vi "ErrorMessage.vi"(0 "VisaCluster":T1, 5 "Message In":string, 11 "error in (no error)":errorcluster) -> (4 "VisaCluster":T1, 6 "Message Out":string, 15 "error out":errorcluster)   [LabVIEW 2014, in "FH 55.lvlib"]
doc: "Dieses VI überprüft die Antwort aus dem Gaussmeter. Ist die Antwort leer oder enthält sie das Wort ERROR wird ein Fehler zurückgegeben.\n\nKeine Antwort: -30000\nERROR:\n parameter: -3999\n command: -4999\n sonstiger: -50000\n\n\n\nThis VI checks the answer from the gaussmeter. If the answer is empty or contains the word ERROR, an error is returned\n\nNo reply -30 000\nERROR:\n Parameters: -3999\n command: -4999\n other: -50 000"
uses:
  FH 55.lvlib
  TypeDef/VisaCluster.ctl
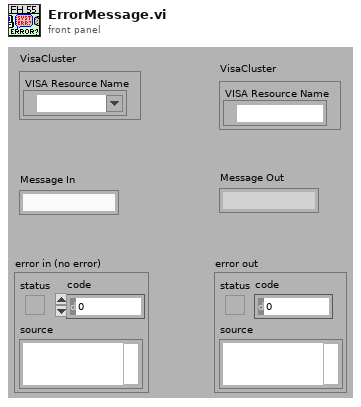
[diagram p1: front panel]
types:
  T1 = typedef "FH 55.lvlib/VisaCluster.ctl" = cluster{"VISA Resource Name":refnum<visa-resource-name>}
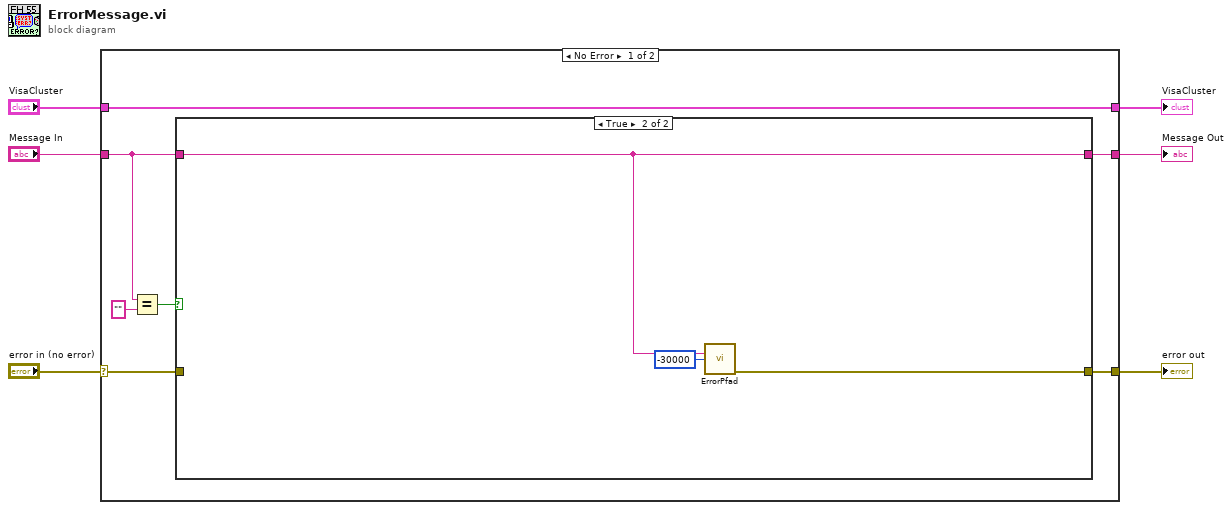
[diagram p0: block diagram]
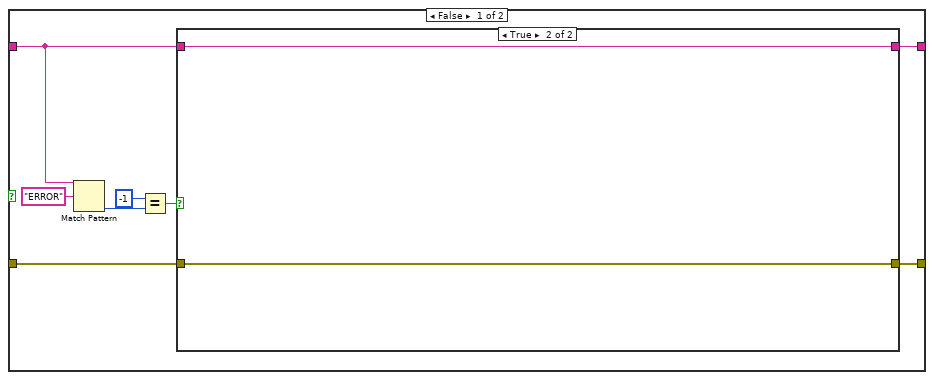
[diagram p2: hidden frame]
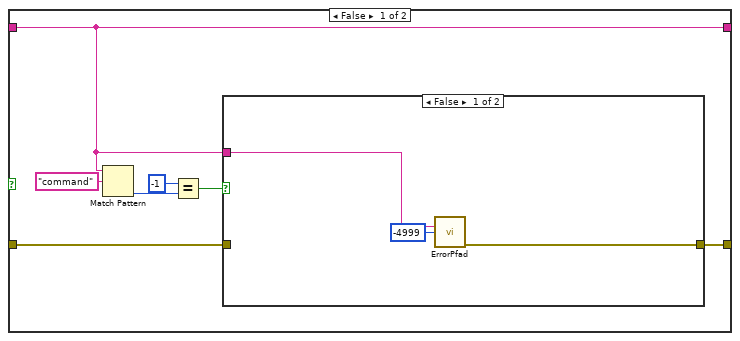
[diagram p3: hidden frame]
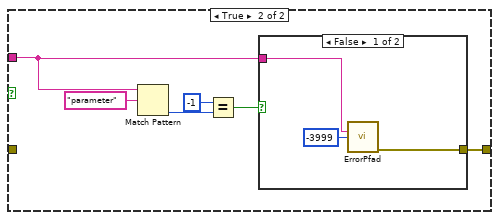
[diagram p4: hidden frame]
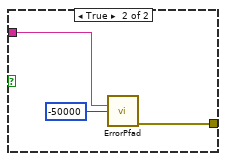
[diagram p5: hidden frame]
diagram:
  n1 = case shown="No Error" "error in (no error)" {
    selector: "error in (no error)" -> [w11 w49]
    tunnel: [w10 w49] -> w5
    tunnel: [w12 w51] -> w3
    tunnel: "VisaCluster" -> [w12 w51]
    tunnel: "Message In" -> [w9 w50]
    tunnel: [w13 w50] -> w1
    frame No Error {
      n2 = Equal?(x=w9, y="") -> (x = y?=w7:bool)
      n3 = case shown="True" w7 {
        tunnel: [w17 w48] -> w13
        tunnel: w11 -> [w16 _]
        tunnel: [w15 w47] -> w10
        tunnel: w9 -> [w14 w48]
        frame False {
          n4 = Match Pattern(string=w14, regular expression="ERROR") -> (offset past match=w20:i32)  [unwired: 1 in, 3 out]
          n5 = Equal?(x=-1, y=w20) -> (x = y?=w18:bool)
          n6 = case shown="True" w18 {
            tunnel: [w23 w44] -> w17
            tunnel: w16 -> [w22 w45]
            tunnel: [w28 w45] -> w15
            tunnel: w14 -> [w23 w44]
            frame False {
              n7 = Match Pattern(string=w23, regular expression="command") -> (offset past match=w26:i32)  [unwired: 1 in, 3 out]
              n8 = Equal?(x=-1, y=w26) -> (x = y?=w24:bool)
              n9 = case shown="False" w24 {
                tunnel: [w29 w32] -> w28
                tunnel: w23 -> [w31 w33]
                tunnel: w22 -> [_ _]
                frame False {
                  n10 = call "ErrorPfad.vi"("Message In"=w31, "Numeric"=-4999 ("code")) -> ("error out"=w29:errorcluster)  [unwired: 12 in, 1 out]
                }
                frame True {
                  n11 = Match Pattern(string=w33, regular expression="parameter") -> (offset past match=w36:i32)  [unwired: 1 in, 3 out]
                  n12 = Equal?(x=-1, y=w36) -> (x = y?=w34:bool)
                  n13 = case shown="False" w34 {
                    tunnel: w33 -> [w39 w42]
                    tunnel: [w38 w41] -> w32
                    frame False {
                      n14 = call "ErrorPfad.vi"("Message In"=w39, "Numeric"=-3999 ("code")) -> ("error out"=w38:errorcluster)  [unwired: 12 in, 1 out]
                    }
                    frame True {
                      n15 = call "ErrorPfad.vi"("Message In"=w42, "Numeric"=-50000 ("code")) -> ("error out"=w41:errorcluster)  [unwired: 12 in, 1 out]
                    }
                  }
                }
              }
            }
            frame True {
            }
          }
        }
        frame True {
          n16 = call "ErrorPfad.vi"("Message In"=w48, "Numeric"=-30000 ("code")) -> ("error out"=w47:errorcluster)  [unwired: 12 in, 1 out]
        }
      }
    }
    frame Error {
    }
  }
  "VisaCluster" <- w3
  "Message Out" <- w1
  "error out" <- w5
